vi "GetODSSpreadsheetData.vi"() -> ()   [LabVIEW 2014]
uses:
  Spreadsheets.ctl
panel:
  out "Table HeaderInfo":string[](array[string])
  out "Header":string="<?xml version=\"1.0\" encoding=\"UTF-8\"?>\n<office:document-content xmlns:office=\"urn:oasis:names:tc:opendocument:xmlns:office:1.0\" xmlns:style=\"urn:oasis:names:tc:opendocument:xmlns:style:1.0\" xmlns:text=\"urn:oasis:names:tc:opendocument:xmlns:text:1.0\" xmlns:table=\"urn:oasis:names:tc:opendocument:xmlns:table:1.0\" xmlns:draw=\"urn:oasis:names:tc:opendocument:xmlns:drawing:1.0\" xmlns:fo=\"urn:oasis:names:tc:opendocument:xmlns:xsl-fo-compatible:1.0\" xmlns:xlink=\"http://www.w3.org/1999/xlink\" xmlns:dc=\"http://purl.org/dc/elements/1.1/\" xmlns:meta=\"urn:oasis:names:tc:opendocument:xmlns:meta:1.0\" xmlns:number=\"urn:oasis:names:tc:opendocument:xmlns:datastyle:1.0\" xmlns:presentation=\"urn:oasis:names:tc:opendocument:xmlns:presentation:1.0\" xmlns:svg=\"urn:oasis:names:tc:opendocument:xmlns:svg-compatible:1.0\" xmlns:chart=\"urn:oasis:names:tc:opendocument:xmlns:chart:1.0\" xmlns:dr3d=\"urn:oasis:names:tc:opendocument:xmlns:dr3d:1.0\" xmlns:math=\"http://www.w3.org/1998/Math/MathML\" xmlns:form=\"urn:oasis:names:tc:opendocument:xmlns:form:1.0\" xmlns:script=\"urn:oasis:names:tc:opendocument:xmlns:script:1.0\" xmlns:ooo=\"http://openoffice.org/2004/office\" xmlns:ooow=\"http://openoffice.org/2004/writer\" xmlns:oooc=\"http://openoffice.org/2004/calc\" xmlns:dom=\"http://www.w3.org/2001/xml-events\" xmlns:xforms=\"http://www.w3.org/2002/xforms\" xmlns:xsd=\"http://www.w3.org/2001/XMLSchema\" xmlns:xsi=\"http://www.w3.org/2001/XMLSchema-instance\" xmlns:rpt=\"http://openoffice.org/2005/report\" xmlns:of=\"urn:oasis:names:tc:opendocument:xmlns:of:1.2\" xmlns:xhtml=\"http://www.w3.org/1999/xhtml\" xmlns:grddl=\"http://www.w3.org/2003/g/data-view#\" xmlns:tableooo=\"http://openoffice.org/2009/table\" xmlns:drawooo=\"http://openoffice.org/2010/draw\" xmlns:calcext=\"urn:org:documentfoundation:names:experimental:calc:xmlns:calcext:1.0\" xmlns:loext=\"urn:org:documentfoundation:names:experimental:office:xmlns:loext:1.0\" xmlns:field=\"urn:openoffice:names:experimental:ooo-ms-interop:xmlns:field:1.0\" xmlns:formx=\"urn:openoffice:names:experimental:ooxml-odf-interop:xmlns:form:1.0\" xmlns:css3t=\"http://www.w3.org/TR/css3-text/\" office:version=\"1.2\"><office:scripts/><office:font-face-decls><style:font-face style:name=\"Liberation Sans\" svg:font-family=\"&apos;Liberation Sans&apos;\" style:font-family-generic=\"swiss\" style:font-pitch=\"variable\"/><style:font-face style:name=\"Mangal\" svg:font-family=\"Mangal\" style:font-family-generic=\"system\" style:font-pitch=\"variable\"/><style:font-face style:name=\"Microsoft YaHei\" svg:font-family=\"&apos;Microsoft YaHei&apos;\" style:font-family-generic=\"system\" style:font-pitch=\"variable\"/><style:font-face style:name=\"Segoe UI\" svg:font-family=\"&apos;Segoe UI&apos;\" style:font-family-generic=\"system\" style:font-pitch=\"variable\"/><style:font-face style:name=\"Tahoma\" svg:font-family=\"Tahoma\" style:font-family-generic=\"system\" style:font-pitch=\"variable\"/></office:font-face-decls><office:automatic-styles><style:style style:name=\"co1\" style:family=\"table-column\"><style:table-column-properties fo:break-before=\"auto\" style:column-width=\"22.58mm\"/></style:style><style:style style:name=\"ro1\" style:family=\"table-row\"><style:table-row-properties style:row-height=\"4.52mm\" fo:break-before=\"auto\" style:use-optimal-row-height=\"true\"/></style:style><style:style style:name=\"ta1\" style:family=\"table\" style:master-page-name=\"Default\"><style:table-properties table:display=\"true\" style:writing-mode=\"lr-tb\"/></style:style></office:automatic-styles><office:body>"
  out "Footer":string="</office:body></office:document-content>"
  in  "archive name":path=path "C:/Users/Steve Watts/Desktop/ISO9000/Checklist/eee - Copy.ods"
  out "Spreadsheet":T1[](array[typedef])
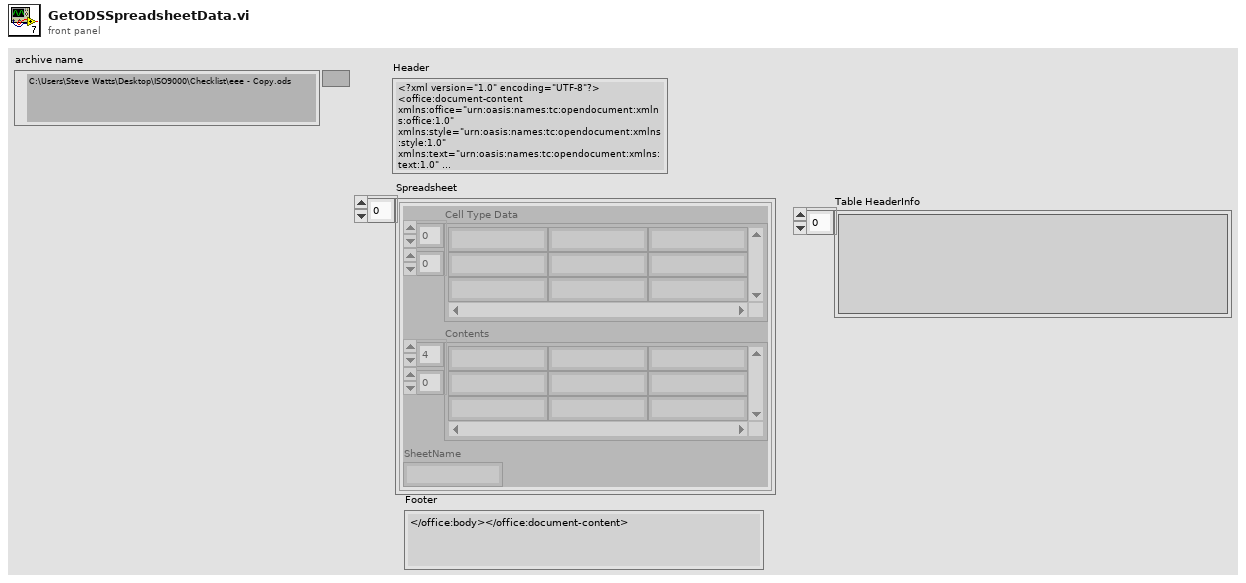
[diagram p1: front panel]
types:
  T1 = typedef "Spreadsheets.ctl" = cluster{"Cell Type Data":string[][], "Contents":string[][], "SheetName":string}
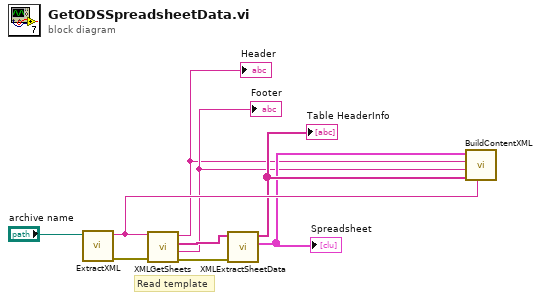
[diagram p0: block diagram]
diagram:
  # "Read template"
  n1 = call "ExtractXML.vi"("archive name"="archive name") -> ("error out"=w8:errorcluster, "byte stream"=w5:string)  [unwired: 9 in]
  n2 = call "XMLGetSheets.vi"("error in (no error)"=w8, "byte stream"=w5) -> ("error out"=w7:errorcluster, "Footer"=w2:string, "Sheets"=w6:string[], "Header"=w1:string)  [unwired: 6 in]
  "Footer" <- w2
  "Header" <- w1
  n3 = call "XMLExtractSheetData.vi"("error in (no error)"=w7, "SheetsXML"=w6) -> ("SpreadsheetData"=w3:T1[], "Table HeaderInfo"=w4:string[])  [unwired: 7 in, 1 out]
  "Spreadsheet" <- w3
  "Table HeaderInfo" <- w4
  n4 = call "BuildContentXML.vi"("Original Content"=w5, "Table HeaderInfo"=w4, "Footer For Spreadsheet"=w2, "Header For Spreadsheet"=w1, "SpreadsheetData"=w3) -> ()  [unwired: 7 in]
